vi "Insert Panel.vi"(8 "error in (no error)":errorcluster, 9 "Index (End)":i32=-1, 10 "Panel In":refnum<class "Panel.lvclass">, 11 "PanelArray in":refnum<class "PanelArray.lvclass">) -> (0 "error out":errorcluster, 3 "PanelArray out":refnum<class "PanelArray.lvclass">)   [LabVIEW 2018, in "OOPanel.lvlib" / "PanelArray.lvclass"]
uses:
  PanelArray.lvclass
  Panel/Panel.lvclass
  PanelArray.lvclass/PanelArray.ctl
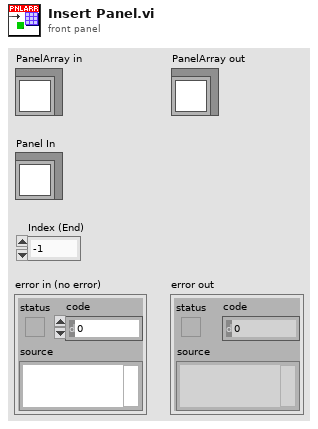
[diagram p1: front panel]
types:
  T1 = typedef "OOPanel.lvlib/PanelArray.lvclass/Ref Data.ctl" = cluster{"State":T2, "Refs":T3, "Events":T4, "Scrolling":T5, "Panels":T6}
  T2 = typedef "OOPanel.lvlib/PanelArray.lvclass/State.ctl" = cluster{"Defer Updates":bool, "Running":bool, "Dynamic Sizing":bool, "Borders":bool}
  T3 = typedef "OOPanel.lvlib/PanelArray.lvclass/Refs.ctl" = cluster{"SubPanels":refnum<vi>[], "Scrollbar":refnum<vi>, "Owning Panel":refnum<vi>}
  T4 = typedef "OOPanel.lvlib/PanelArray.lvclass/Events.ctl" = cluster{"Close":refnum<user-event>}
  T5 = typedef "OOPanel.lvlib/PanelArray.lvclass/Scrolling.ctl" = cluster{"Size":i32, "Max":i32, "Current":i32, "Top Index":i32, "Heights":i32[]}
  T6 = typedef "OOPanel.lvlib/PanelArray.lvclass/Panels.ctl" = cluster{"All":refnum<class "Panel.lvclass">[], "Visible":refnum<class "Panel.lvclass">[], "Blank":refnum<class "ArrayBlank.lvclass">}
  T7 = typedef "OOPanel.lvlib/Panel.lvclass/Desired Size.ctl" = cluster{"Width":i16, "Height":i16}
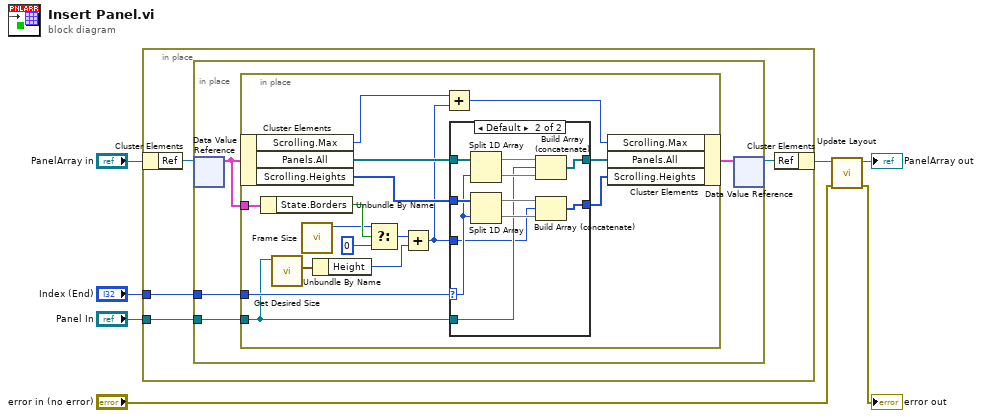
[diagram p0: block diagram]
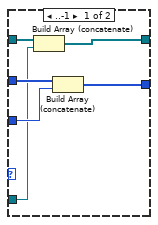
[diagram p2: hidden frame]
diagram:
  n1 = in-place {
    in-place-border: "Index (End)" -> [w11]
    in-place-border: "Panel In" -> [w10]
    n2 = in-place-cluster #1("PanelArray in") -> ("Ref"=w9:refnum<data-value>)
    n3 = in-place {
      in-place-border: w11 -> [w15]
      in-place-border: w10 -> [w14]
      n4 = in-place-dvr #2(w9) -> (w12:T1)  [unwired: 1 out]
      n5 = in-place {
        in-place-border: w15 -> [w30]
        in-place-border: w14 -> [w22]
        in-place-border: w12 -> [w24]
        n6 = in-place-cluster #3(w12) -> ("Scrolling.Max"=w26:i32, "Panels.All"=w31:refnum<class "Panel.lvclass">[], "Scrolling.Heights"=w28:i32[])
        n7 = Unbundle By Name(w24) -> ("State.Borders"=w21:bool)
        n8 = call-dynamic "Get Desired Size.vi"("Panel in"=w22) -> ("Desired Size"=w23:T7)  [unwired: 8 in, 2 out]
        n9 = call "Frame Size.vi"() -> ("Frame Size"=w16:i32)  [unwired: 11 in]
        n10 = Unbundle By Name(w23) -> ("Height"=w19:i16)
        n11 = Select(t=w16, s=w21, f=0) -> (s? t:f=w18:i32)
        n12 = Add(x=w18, y=w19) -> (x+y=w17:i32)
        n13 = Add(x=w26, y=w17) -> (x+y=w25:i32)
        n14 = case shown="Default" w30 {
          selector: w30 -> [_ w41]
          tunnel: w31 -> [w37 w48]
          tunnel: w22 -> [w32 w39]
          tunnel: [w36 w45] -> w29
          tunnel: w28 -> [w35 w42]
          tunnel: [w34 w40] -> w27
          tunnel: w17 -> [w33 w38]
          frame ..-1 {
            n15 = Build Array (concatenate)(w37, w32) -> (w36:refnum<class "Panel.lvclass">[])
            n16 = Build Array (concatenate)(w35, w33) -> (w34:i32[])
          }
          frame Default {
            n17 = Split 1D Array(array=w48, index=w41) -> (first subarray=w47:refnum<class "Panel.lvclass">[], second subarray=w46:refnum<class "Panel.lvclass">[])
            n18 = Split 1D Array(array=w42, index=w41) -> (first subarray=w43:i32[], second subarray=w44:i32[])
            n19 = Build Array (concatenate)(w47, w39, w46) -> (w45:refnum<class "Panel.lvclass">[])
            n20 = Build Array (concatenate)(w43, w38, w44) -> (w40:i32[])
          }
        }
        n21 = in-place-cluster #3("Scrolling.Max"=w25, "Panels.All"=w29, "Scrolling.Heights"=w27) -> (w13:T1)
      }
      n22 = in-place-dvr #2(w13) -> (w8:refnum<data-value>)  [unwired: 1 out]
    }
    n23 = in-place-cluster #1("Ref"=w8) -> (w5:refnum<class "PanelArray.lvclass">)
  }
  n24 = call "Update Layout.vi"("error in (no error)"="error in (no error)", "PanelArray in"=w5) -> ("error out"=→"error out":errorcluster, "PanelArray out"=→"PanelArray out":refnum<class "PanelArray.lvclass">)  [unwired: 8 in]
